vi "PictureSelector.vi"(8 "Input Selection 2":i32, 9 "Input Picture 2":picture, 10 "Input Selection 1":i32, 11 "Input Picture 1":picture) -> (0 "Output Selection 2":i32, 1 "Output picture 2":picture, 2 "Output Selection 1":i32, 3 "Output picture":picture, 5 "Error":bool)   [LabVIEW 2021]
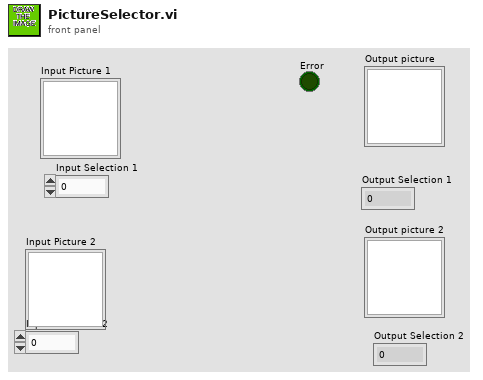
[diagram p1: front panel]
types:
  T1 = typedef "imagedata.ctl" = cluster{"image type":i32, "image depth":i32, "image":u8[], "mask":u8[], "colors":u32[], "Rectangle":cluster{"left":i16, "top":i16, "right":i16, "bottom":i16}}
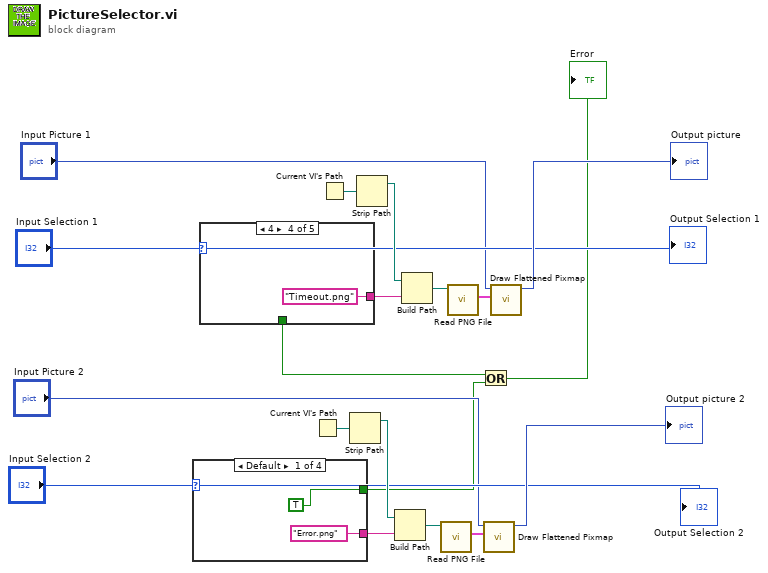
[diagram p0: block diagram]
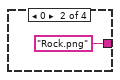
[diagram p2: hidden frame]
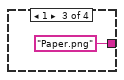
[diagram p3: hidden frame]
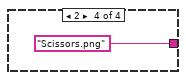
[diagram p4: hidden frame]
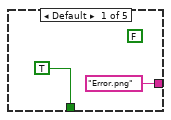
[diagram p5: hidden frame]
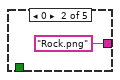
[diagram p6: hidden frame]
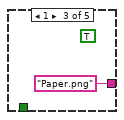
[diagram p7: hidden frame]
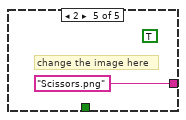
[diagram p8: hidden frame]
diagram:
  n1 = case shown="Default" "Input Selection 2" {
    tunnel: ["Error.png" ("String 2") "Rock.png" ("String 2") "Paper.png" ("String 2") "Scissors.png" ("String 2")] -> w11
    tunnel: [TRUE _ _ _] -> w2
    frame Default {
    }
    frame 0 {
    }
    frame 1 {
    }
    frame 2 {
    }
  }
  n2 = case shown="4" "Input Selection 1" {
    tunnel: ["Error.png" ("String 2") "Rock.png" ("String 2") "Paper.png" ("String 2") "Timeout.png" ("String 2") "Scissors.png" ("String 2")] -> w19
    tunnel: [TRUE _ _ _ _] -> w3
    frame Default {
      (unwired) FALSE ("stop")
    }
    frame 0 {
    }
    frame 1 {
      (unwired) TRUE ("stop")
    }
    frame 4 {
    }
    frame 2 {
      (unwired) TRUE ("stop")
      # "change the image here"
    }
  }
  n3 = Current VI's Path() -> (path=w8:path)
  n4 = Current VI's Path() -> (path=w16:path)
  n5 = Strip Path(path=w8) -> (stripped path=w10:path)  [unwired: 1 out]
  n6 = Strip Path(path=w16) -> (stripped path=w18:path)  [unwired: 1 out]
  n7 = Build Path(base path=w10, name or relative path=w11) -> (appended path=w9:path)
  n8 = Build Path(base path=w18, name or relative path=w19) -> (appended path=w17:path)
  n9 = call <vilib>:"Read PNG File.vi"("path to PNG file"=w9) -> ("image data"=w7:T1)  [unwired: 8 in, 2 out]
  n10 = call <vilib>:"Read PNG File.vi"("path to PNG file"=w17) -> ("image data"=w15:T1)  [unwired: 8 in, 2 out]
  n11 = Or(x=w3, y=w2) -> (x .or. y?=→"Error":bool)
  n12 = call <vilib>:"Draw Flattened Pixmap.vi"("image data"=w7, "picture"="Input Picture 2") -> ("new picture"=→"Output picture 2":picture)  [unwired: 7 in]
  n13 = call <vilib>:"Draw Flattened Pixmap.vi"("image data"=w15, "picture"="Input Picture 1") -> ("new picture"=→"Output picture":picture)  [unwired: 7 in]
  "Output Selection 1" <- "Input Selection 1"
  "Output Selection 2" <- "Input Selection 2"
